vi "initialize_arduinos_subVI.vi"(10 "arduino 1-6 addresses":T2, 11 "arduinos on?":bool) -> (1 "arduino addresses/errors":T1, 3 "arduinos on/off":bool)   [LabVIEW 2014]
uses:
  <vilib>/Instr/_visa.llb/VISA Configure Serial Port (Instr).vi
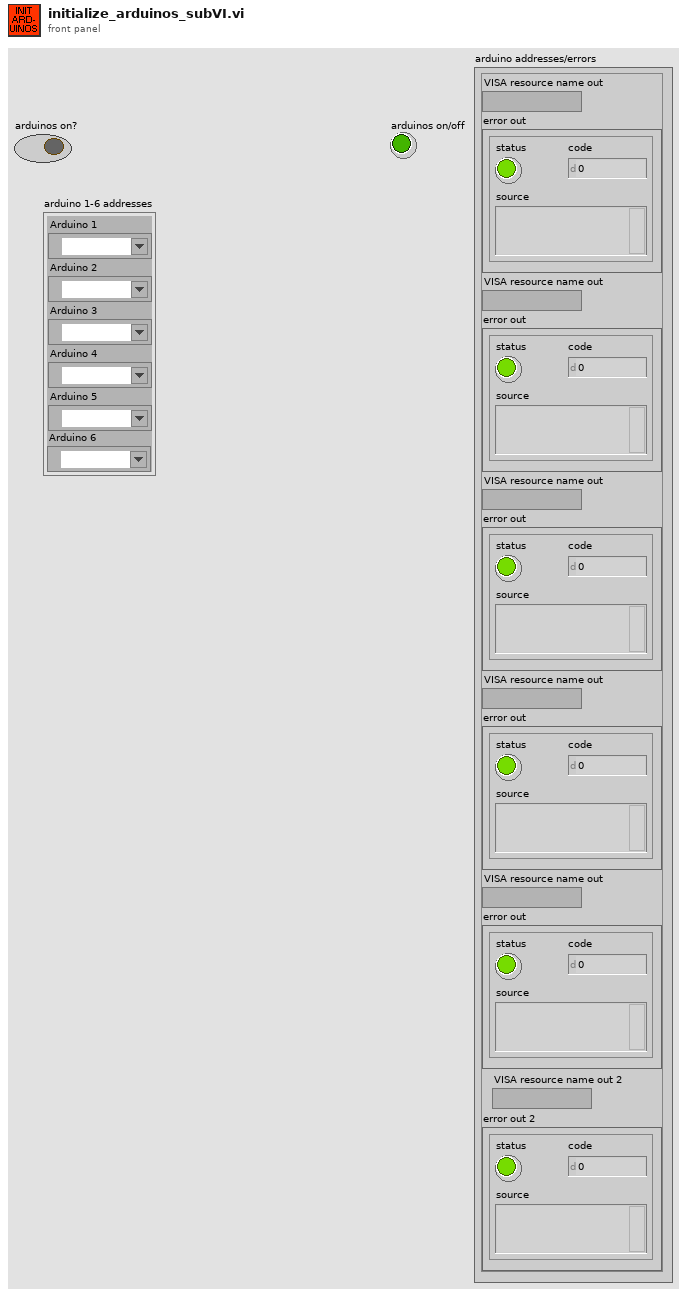
[diagram p1: front panel]
types:
  T1 = cluster{"VISA resource name out":refnum<visa-resource-name>, "error out":errorcluster, "VISA resource name out":refnum<visa-resource-name>, "error out":errorcluster, "VISA resource name out":refnum<visa-resource-name>, "error out":errorcluster, "VISA resource name out":refnum<visa-resource-name>, "error out":errorcluster, "VISA resource name out":refnum<visa-resource-name>, "error out":errorcluster, "VISA resource name out 2":refnum<visa-resource-name>, "error out 2":errorcluster}
  T2 = cluster{"Arduino 1":refnum<visa-resource-name>, "Arduino 2":refnum<visa-resource-name>, "Arduino 3":refnum<visa-resource-name>, "Arduino 4":refnum<visa-resource-name>, "Arduino 5":refnum<visa-resource-name>, "Arduino 6":refnum<visa-resource-name>}
  T3 = cluster{"VISA resource name out":refnum<visa-resource-name>, "error out":errorcluster, "VISA resource name out":refnum<visa-resource-name>, "error out":errorcluster, "VISA resource name out":refnum<visa-resource-name>, "error out":errorcluster, "VISA resource name out":refnum<visa-resource-name>, "error out":errorcluster, "VISA resource name out":refnum<visa-resource-name>, "error out":errorcluster, "VISA resource name out":refnum<visa-resource-name>, "error out":errorcluster}
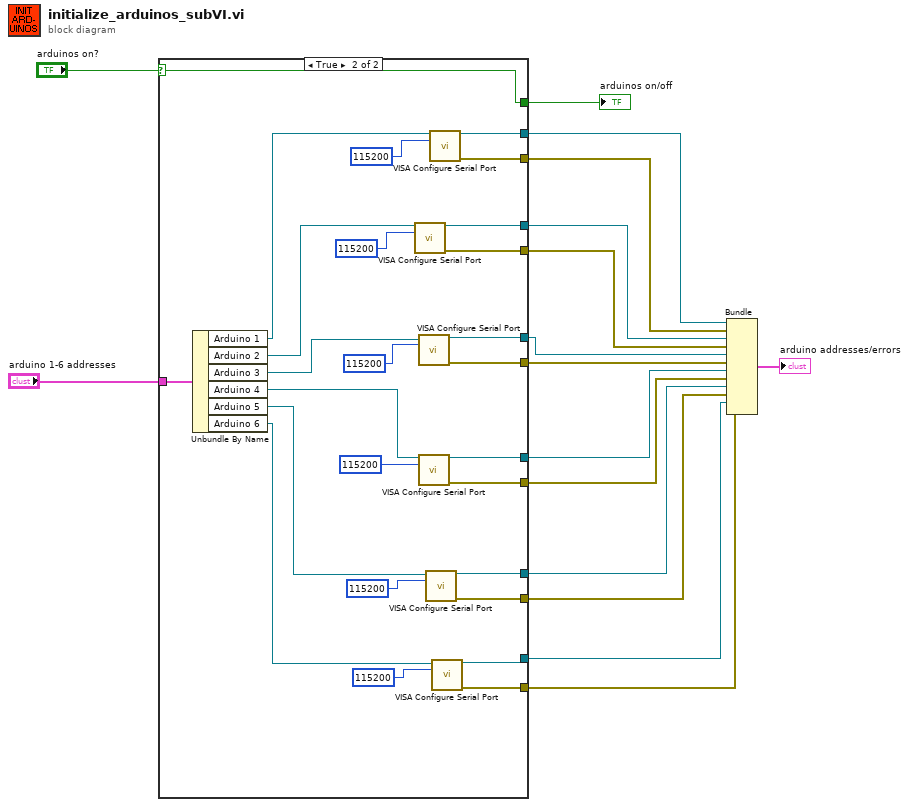
[diagram p0: block diagram]
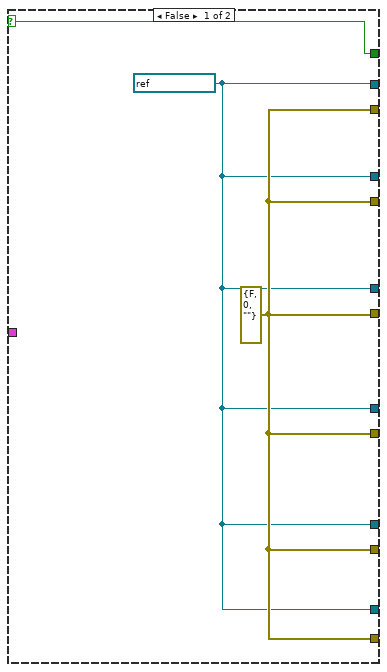
[diagram p2: hidden frame]
diagram:
  n1 = case shown="True" "arduinos on?" {
    selector: "arduinos on?" -> [w19 w45]
    tunnel: [w19 w45] -> w15
    tunnel: [w17 w43] -> w13
    tunnel: [w18 w42] -> w12
    tunnel: [w17 w40] -> w11
    tunnel: [w18 w39] -> w10
    tunnel: [w17 w37] -> w9
    tunnel: [w18 w36] -> w8
    tunnel: [w17 w33] -> w7
    tunnel: [w18 w32] -> w6
    tunnel: [w17 w31] -> w5
    tunnel: [w18 w30] -> w4
    tunnel: "arduino 1-6 addresses" -> [_ w26]
    tunnel: [w17 w28] -> w2
    tunnel: [w18 w27] -> w1
    frame False {
      w18 = errorcluster {"status"=FALSE, "code"=0, "source"=""} ("error out")
      w17 = refnum<visa-resource-name> refnum ("VISA resource name out")
    }
    frame True {
      n2 = Unbundle By Name(w26) -> ("Arduino 1"=w25:refnum<visa-resource-name>, "Arduino 2"=w24:refnum<visa-resource-name>, "Arduino 3"=w23:refnum<visa-resource-name>, "Arduino 4"=w22:refnum<visa-resource-name>, "Arduino 5"=w21:refnum<visa-resource-name>, "Arduino 6"=w20:refnum<visa-resource-name>)
      n3 = call-poly "VISA Configure Serial Port"("VISA resource name"=w24, "baud rate (9600)"=u32 115200) -> ("VISA resource name out"=w40:refnum<visa-resource-name>, "error out"=w39:errorcluster)  [unwired: 12 in]
      n4 = call-poly "VISA Configure Serial Port"("VISA resource name"=w23, "baud rate (9600)"=u32 115200) -> ("VISA resource name out"=w37:refnum<visa-resource-name>, "error out"=w36:errorcluster)  [unwired: 12 in]
      n5 = call-poly "VISA Configure Serial Port"("VISA resource name"=w22, "baud rate (9600)"=u32 115200) -> ("VISA resource name out"=w33:refnum<visa-resource-name>, "error out"=w32:errorcluster)  [unwired: 12 in]
      n6 = call-poly "VISA Configure Serial Port"("VISA resource name"=w21, "baud rate (9600)"=u32 115200) -> ("VISA resource name out"=w31:refnum<visa-resource-name>, "error out"=w30:errorcluster)  [unwired: 12 in]
      n7 = call-poly "VISA Configure Serial Port"("VISA resource name"=w25, "baud rate (9600)"=u32 115200) -> ("VISA resource name out"=w43:refnum<visa-resource-name>, "error out"=w42:errorcluster)  [unwired: 12 in]
      n8 = call-poly "VISA Configure Serial Port"("VISA resource name"=w20, "baud rate (9600)"=u32 115200) -> ("VISA resource name out"=w28:refnum<visa-resource-name>, "error out"=w27:errorcluster)  [unwired: 12 in]
    }
  }
  "arduinos on/off" <- w15
  n9 = Bundle("VISA resource name out"=w13, "error out"=w12, "VISA resource name out"=w11, "error out"=w10, "VISA resource name out"=w9, "error out"=w8, "VISA resource name out"=w7, "error out"=w6, "VISA resource name out"=w5, "error out"=w4, "VISA resource name out"=w2, "error out"=w1) -> (→"arduino addresses/errors":T3)  [unwired: 1 in]
